vi "Get Raw Key Value Array.vi"(0 "DBMap in":refnum<class "DBMap.lvclass">, 11 "error in (no error)":errorcluster {"code" format="Error %.0f"}) -> (4 "DBMap out":refnum<class "DBMap.lvclass">, 6 "KV Array Raw":string[][](table) caption="Result Set (from first statement with results)", 15 "error out":errorcluster {"code" format="Error %.0f"})   [LabVIEW 2020, in "DBMap.lvclass"]
uses:
  DBMap.lvclass
  DBMap.lvclass/DBMap.ctl
  <vilib>/drjdpowell/SQLite Library/SQLite.lvlib
  <vilib>/drjdpowell/SQLite Library/SQL Connection/Execute SQL.vi
  <vilib>/drjdpowell/SQLite Library/SQL Connection/Connection.lvclass
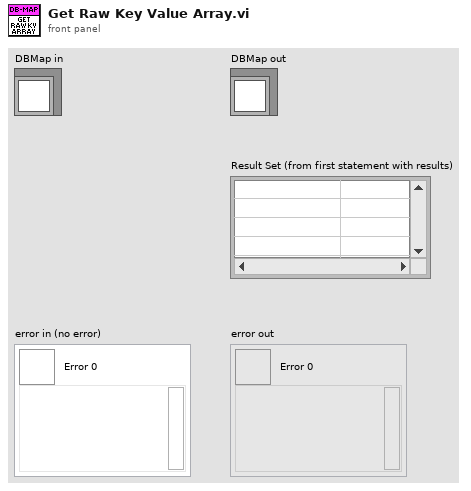
[diagram p1: front panel]
types:
  T1 = typedef "Semaphore RefNum" = refnum<k1>
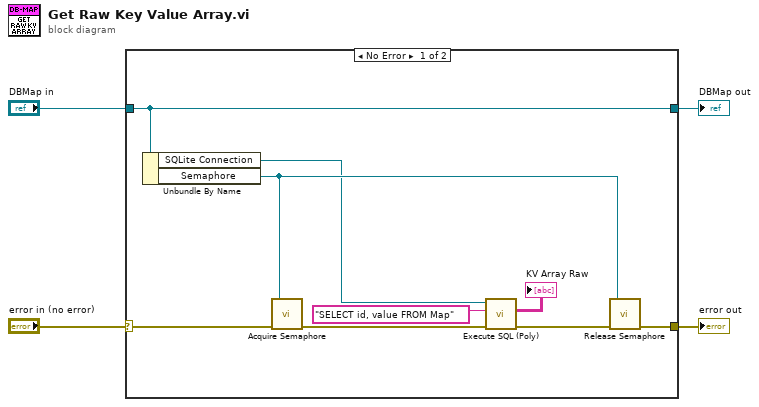
[diagram p0: block diagram]
diagram:
  n1 = case shown="No Error" "error in (no error)" {
    selector: "error in (no error)" -> [w12 w15]
    tunnel: [w11 w15] -> w3
    tunnel: [w13 w14] -> w1
    tunnel: "DBMap in" -> [w13 w14]
    frame No Error {
      n2 = Unbundle By Name(w13) -> ("SQLite Connection"=w7:refnum<class "Connection.lvclass">, "Semaphore"=w10:T1)
      n3 = call <vilib>:"Acquire Semaphore.vi"("error in (no error)"=w12, "semaphore"=w10) -> ("error out"=w8:errorcluster)  [unwired: 3 in, 2 out]
      n4 = call-poly <vilib>:"Execute SQL (Poly).vi"("error in (no error)"=w8, "SQL"="SELECT id, value FROM Map", "SQLite Connection in"=w7) -> ("error out"=w6:errorcluster, "Result Set"=→"KV Array Raw":string[][])  [unwired: 5 in, 2 out]
      n5 = call <vilib>:"Release Semaphore.vi"("error in (no error)"=w6, "semaphore"=w10) -> ("error out"=w11:errorcluster)  [unwired: 4 in, 1 out]
    }
    frame Error {
    }
  }
  "error out" <- w3
  "DBMap out" <- w1
